vi "Get Number New Images.vi"(8 "error in (no error)":errorcluster, 11 "CCDCamera in":refnum<class "Simulated_CCD_Camera.lvclass">) -> (0 "error out":errorcluster, 2 "New Images ?":bool, 3 "CCDCamera out":refnum<class "Simulated_CCD_Camera.lvclass">)   [LabVIEW 2018, in "Simulated_CCD_Camera.lvclass"]
uses:
  Simulated_CCD_Camera.lvclass
  Simulated_CCD_Camera.lvclass/Simulated_CCD_Camera.ctl
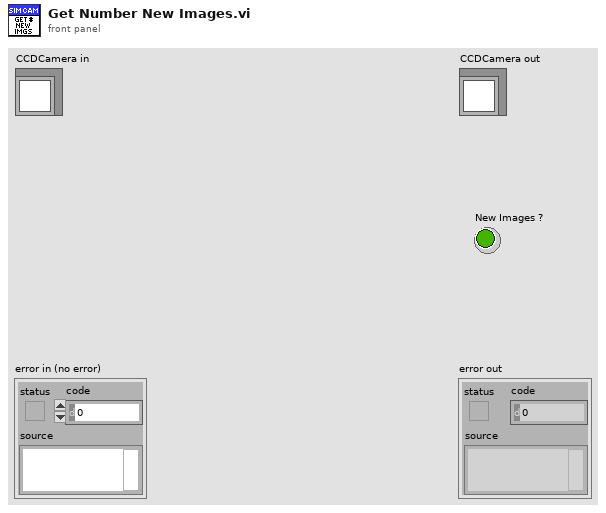
[diagram p1: front panel]
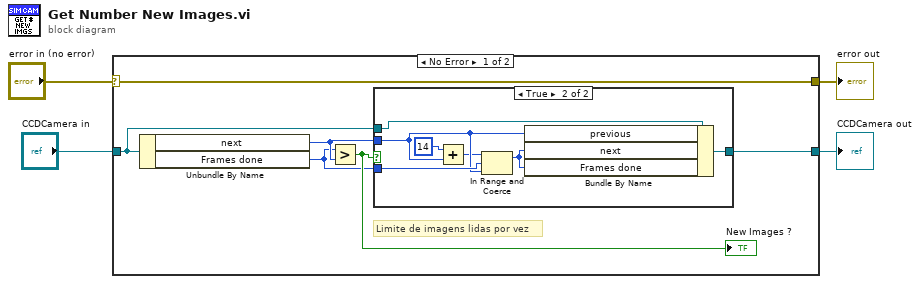
[diagram p0: block diagram]
diagram:
  n1 = case shown="No Error" "error in (no error)" {
    selector: "error in (no error)" -> [w10 w20]
    tunnel: [w10 w20] -> w3
    tunnel: [w9 w19] -> w1
    tunnel: "CCDCamera in" -> [w8 w19]
    frame No Error {
      # "Limite de imagens lidas por vez"
      n2 = Unbundle By Name(w8) -> ("next"=w6:u16, "Frames done"=w5:u32)
      n3 = Greater?(x=w5, y=w6) -> (0:w7:bool)
      "New Images ?" <- w7
      n4 = case shown="True" w7 {
        tunnel: [w11 w18] -> w9
        tunnel: w8 -> [w11 w17]
        tunnel: w5 -> [_ w16]
        tunnel: w6 -> [_ w15]
        frame False {
        }
        frame True {
          n5 = Add(x=u16 14, y=w15) -> (x+y=w14:u16)
          n6 = In Range and Coerce(upper limit=w14, x=w16, lower limit=w15) -> (coerced(x)=w12:u32)  [unwired: 1 out]
          n7 = Bundle By Name(cluster=w17, "previous"=w15, "next"=w12, "Frames done"=w12) -> (w18:refnum<class "Simulated_CCD_Camera.lvclass">)
        }
      }
    }
    frame Error {
    }
  }
  "error out" <- w3
  "CCDCamera out" <- w1
